vi "数组大小.vi"() -> ()   [LabVIEW 2012]
panel:
  out "大小 2":i32[](array[numeric])
  out "大小":i32
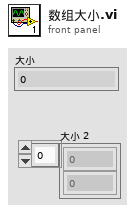
[diagram p1: front panel]
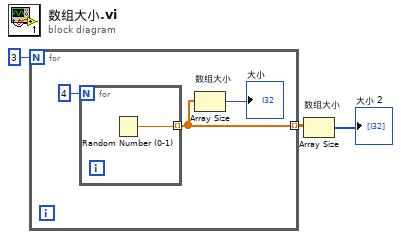
[diagram p0: block diagram]
diagram:
  n1 = for {
    N: 3 -> [_]
    tunnel: [w5] -> w2 mode=indexing
    n2 = for {
      N: 4 -> [_]
      tunnel: [w7] -> w5 mode=indexing
      n3 = Random Number (0-1)() -> (number: 0 to 1=w7:dbl)
    }
    n4 = Array Size "数组大小"(array=w5) -> (size(s)=→"大小":i32)
  }
  n5 = Array Size "数组大小"(array=w2) -> (size(s)=→"大小 2":i32[])
